vi "호출자(엄격하지않은).vi"() -> ()   [LabVIEW 2014]
panel:
  out "웨이브폼 그래프":cluster{"f0":dbl, "df":dbl, "magnitude":dbl[]}(graph)
  in  "frequency":dbl=100.0
  in  "signal type":T1(ring)
  out "에러 출력":errorcluster
  in  "vi 경로":path=path "C:/Users/LVEDU09/Documents/YSK/호출대상.vi"
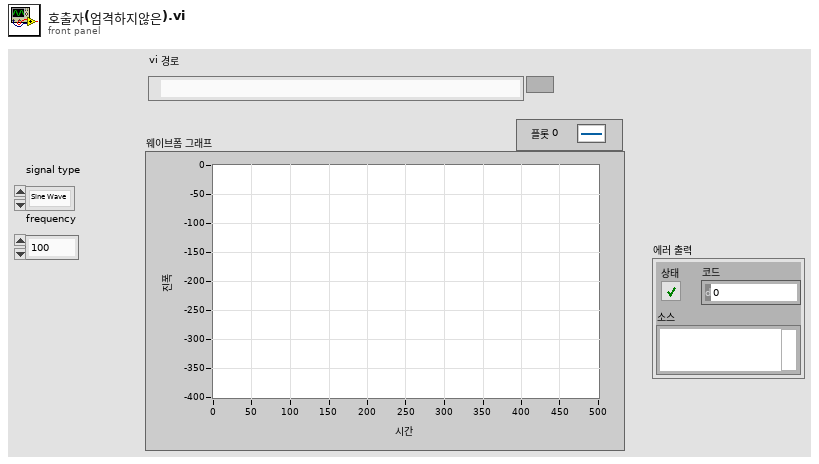
[diagram p1: front panel]
types:
  T1 = enum16{"Sine Wave", "Triangle Wave", "Square Wave", "Sawtooth Wave"}
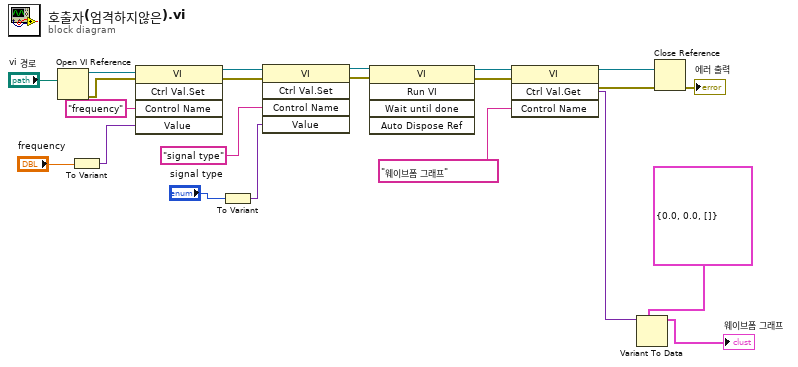
[diagram p0: block diagram]
diagram:
  n1 = Open VI Reference(vi path="vi 경로") -> (vi reference=w18:refnum<vi>, error out=w15:errorcluster)  [unwired: 5 in]
  n2 = To Variant(anything="frequency") -> (Variant=w8:variant)
  n3 = invoke class="VI" method="Ctrl Val.Set"(reference=w18, error in=w15, "Control Name"="frequency" ("컨트롤 이름"), "Value"=w8) -> (reference out=w13:refnum<vi>, error out=w14:errorcluster)  [unwired: 1 in, 3 out]
  n4 = To Variant(anything="signal type") -> (Variant=w5:variant)
  n5 = invoke class="VI" method="Ctrl Val.Set"(reference=w13, error in=w14, "Control Name"="signal type" ("컨트롤 이름"), "Value"=w5) -> (reference out=w17:refnum<vi>, error out=w12:errorcluster)  [unwired: 1 in, 3 out]
  n6 = invoke class="VI" method="Run VI"(reference=w17, error in=w12) -> (reference out=w16:refnum<vi>, error out=w11:errorcluster)  [unwired: 3 in, 3 out]
  n7 = invoke class="VI" method="Ctrl Val.Get"(reference=w16, error in=w11, "Control Name"="웨이브폼 그래프" ("컨트롤 이름")) -> (reference out=w20:refnum<vi>, error out=w19:errorcluster, "Get Control Value Variant"=w3:variant)  [unwired: 1 in, 1 out]
  n8 = Variant To Data(type=cluster{dbl, dbl, dbl[]} {0.0, 0.0, []}, Variant=w3) -> (data=→"웨이브폼 그래프":cluster{dbl, dbl, dbl[]})  [unwired: 1 in, 1 out]
  n9 = Close Reference(reference=w20, error in (no error)=w19) -> (error out=→"에러 출력":errorcluster)
